vi "ble_scan_parameters.vi"(6 "Scanning Technique":T1=1 items=["Pasive", "Active"], 8 "error in (no error)":errorcluster, 9 "Scan Window (125ms)":u16=125, 10 "Scan Interval (125ms)":u16=125, 11 "COM Bluegiga in":refnum<visa-resource-name>) -> (0 "error out":errorcluster, 2 "success?":bool, 3 "COM Bluegiga out":refnum<visa-resource-name>)   [LabVIEW 2015]
uses:
  type_def/scanning_technique.ctl
panel:
  out "full message package":u8[](array[numeric])
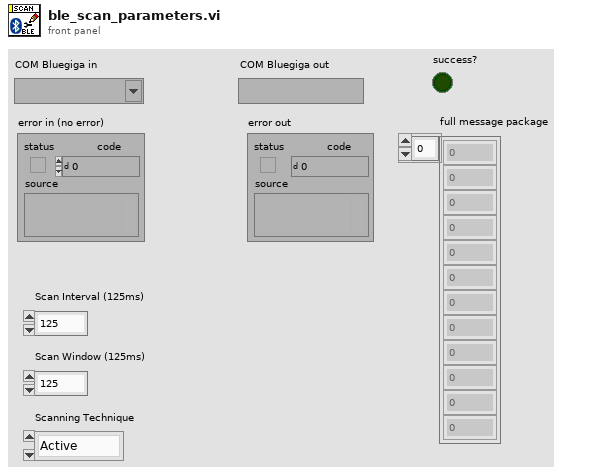
[diagram p1: front panel]
types:
  T1 = typedef "scanning_technique.ctl" = u8
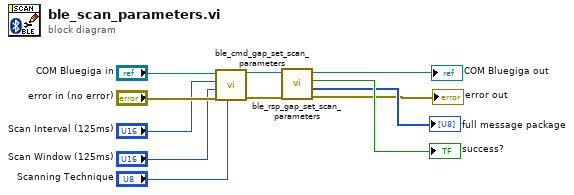
[diagram p0: block diagram]
diagram:
  n1 = call "ble_cmd_gap_set_scan_parameters.vi"("Scanning Technique"="Scanning Technique", "error in (no error)"="error in (no error)", "Scan Window (125ms)"="Scan Window (125ms)", "Scan Interval (125ms)"="Scan Interval (125ms)", "COM Bluegiga in"="COM Bluegiga in") -> ("error out"=w6:errorcluster, "COM Bluegiga out"=w5:refnum<visa-resource-name>)  [unwired: 5 in]
  n2 = call "ble_rsp_gap_set_scan_parameters.vi"("error in (no error)"=w6, "COM Bluegiga in"=w5) -> ("error out"=→"error out":errorcluster, "full message package"=→"full message package":u8[], "success?"=→"success?":bool, "COM Bluegiga out"=→"COM Bluegiga out":refnum<visa-resource-name>)  [unwired: 6 in]
